vi "电阻应变_5.vi"(0 "R0-1":dbl, 1 "R0-2":dbl, 2 "温度":dbl=100.0 format="%#_13g", 3 "SL1":dbl, 4 "SL1 2":dbl, 5 "L 1":dbl, 6 "L 2":dbl) -> (7 "strain1":dbl, 8 "strain 2":dbl)   [LabVIEW 2019]
panel:
  out "补偿电阻 1":dbl format="%#_10g"
  out "补偿电阻 2":dbl format="%#.8g"
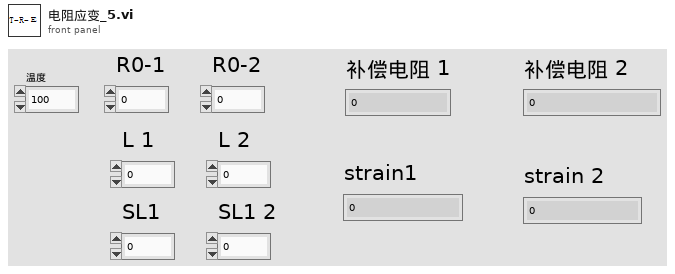
[diagram p1: front panel]
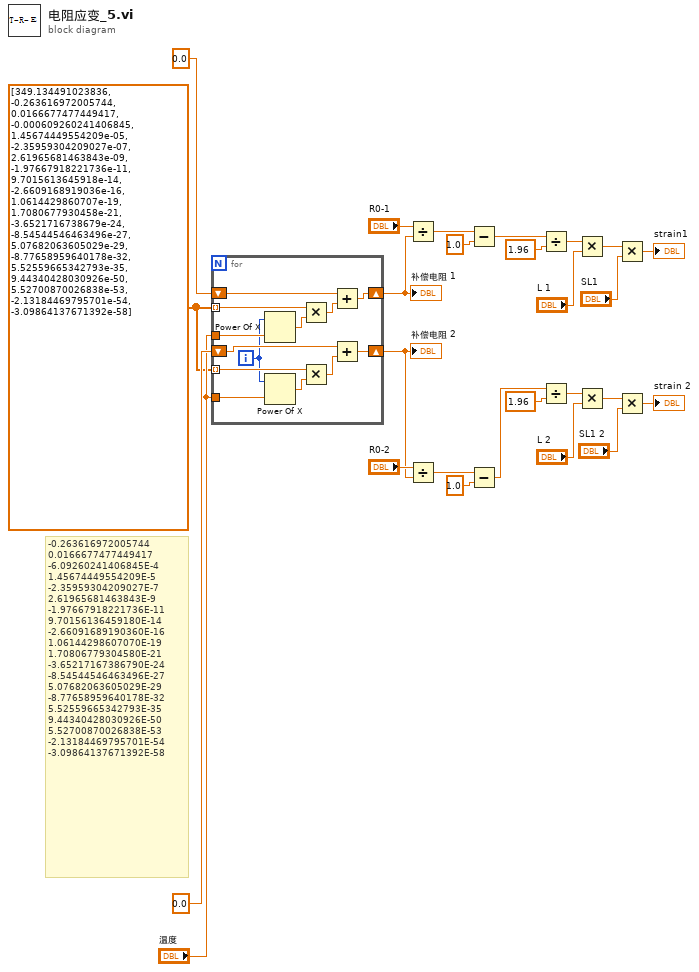
[diagram p0: block diagram]
diagram:
  w1 = dbl[] [349.134491023836, -0.263616972005744, 0.0166677477449417, -0.000609260241406845, 1.45674449554209e-05, -2.35959304209027e-07, 2.61965681463843e-09, -1.97667918221736e-11, 9.7015613645918e-14, -2.6609168919036e-16, 1.0614429860707e-19, 1.7080677930458e-21, -3.6521716738679e-24, -8.54544546463496e-27, 5.07682063605029e-29, -8.77658959640178e-32, 5.52559665342793e-35, 9.44340428030926e-50, 5.52700870026838e-53, -2.13184469795701e-54, -3.09864137671392e-58] ("Array")
  # "-0.263616972005744\n0.0166677477449417\n-6.09260241406845E-4\n1.45674449554209E-5\n-2.35959304209027E-7\n2.61965681463843E-9\n-1.97667918221736E-11\n9.70156136459180E-14\n-2.66091689190360E-16\n1.06144298607070E-19\n1.70806779304580E-21\n-3.65217167386790E-24\n-8.54544546463496E-27\n5.07682063605029E-29\n-8.77658959640178E-32\n5.52559665342793E-35\n9.44340428030926E-50\n5.52700870026838E-53\n-2.13184469795701E-54\n-3.09864137671392E-58"
  n1 = for {
    tunnel: w1 -> [w39] mode=indexing
    tunnel: "温度" -> [w38]
    shift-right: [w37] -> w21
    shift-left: 0.0 -> [w36]
    shift-right: [w31] -> w14
    shift-left: 0.0 -> [w32]
    tunnel: w1 -> [w30] mode=indexing
    tunnel: "温度" -> [w29]
    i -> [w28]
    n2 = Power Of X(1:w29, 2:w28) -> (0:w34:dbl)
    n3 = Power Of X(1:w38, 2:w28) -> (0:w35:dbl)
    n4 = Multiply(x=w30, y=w34) -> (x*y=w33:dbl)
    n5 = Multiply(x=w39, y=w35) -> (x*y=w27:dbl)
    n6 = Add(x=w32, y=w33) -> (x+y=w31:dbl)
    n7 = Add(x=w36, y=w27) -> (x+y=w37:dbl)
  }
  "补偿电阻 2" <- w21
  "补偿电阻 1" <- w14
  n8 = Divide(x="R0-1", y=w14) -> (x/y=w17:dbl)
  n9 = Divide(x="R0-2", y=w21) -> (x/y=w20:dbl)
  n10 = Subtract(x=w17, y=1.0) -> (x-y=w13:dbl)
  n11 = Subtract(x=w20, y=1.0) -> (x-y=w18:dbl)
  n12 = Divide(x=w13, y=1.96) -> (x/y=w12:dbl)
  n13 = Divide(x=w18, y=1.96) -> (x/y=w10:dbl)
  n14 = Multiply(x=w12, y="L 1") -> (x*y=w8:dbl)
  n15 = Multiply(x=w10, y="L 2") -> (x*y=w6:dbl)
  n16 = Multiply(x=w8, y="SL1") -> (x*y=→"strain1":dbl)
  n17 = Multiply(x=w6, y="SL1 2") -> (x*y=→"strain 2":dbl)
